vi "Command (read) - RL.vi"(7 "timeout ms (100)":i32=100, 8 "error in (no error)":errorcluster, 9 "Register":string, 10 "IP":string, 11 "connection ID in":refnum<k16>) -> (0 "error out":errorcluster, 2 "Register Value":string, 3 "connection ID out":refnum<k16>)   [LabVIEW 2016, in "SMD-7615.lvlib" / "eSCL.lvlib"]
doc: "RL - Register Load - immediate\nSets a data register to the given immediate data value. The data value is checked and stored as a Long word. When setting a Short-word register with the given Long-word data value only the lower word of the Long value is used."
uses:
  eSCL.lvlib
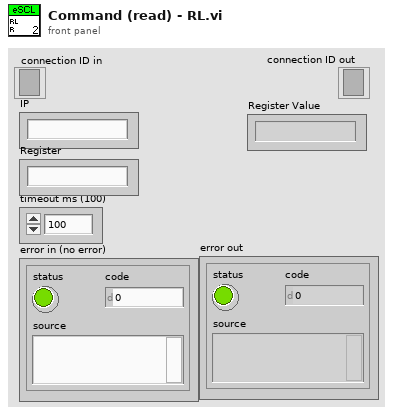
[diagram p1: front panel]
types:
  T1 = typedef "SMD-7615.lvlib/eSCL.lvlib/UDP Received Data.ctl" = cluster{"Received String":string, "eSCL Cmd":string, "Data":string}
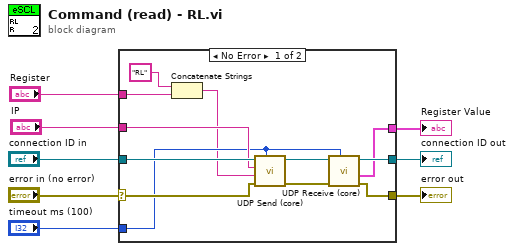
[diagram p0: block diagram]
diagram:
  n1 = case shown="No Error" "error in (no error)" {
    selector: "error in (no error)" -> [w16 w21]
    tunnel: "connection ID in" -> [w15 w22]
    tunnel: [w18 w22] -> w6
    tunnel: [w17 w21] -> w5
    tunnel: "IP" -> [w14 _]
    tunnel: "timeout ms (100)" -> [w13 _]
    tunnel: [w9 _] -> w2
    tunnel: "Register" -> [w11 _]
    frame No Error {
      n2 = Concatenate Strings("RL" ("Data"), w11) -> (w10:string)
      n3 = call "UDP Send (core).vi"("timeout ms (100)"=w13, "error in (no error)"=w16, "Data"=w10, "IP"=w14, "connection ID in"=w15) -> ("error out"=w20:errorcluster, "connection ID out"=w19:refnum<k16>)  [unwired: 5 in]
      n4 = call "UDP Receive (core).vi"("timeout ms (100)"=w13, "error in (no error)"=w20, "connection ID in"=w19) -> ("error out"=w17:errorcluster, "Received Data"=w9:T1, "connection ID out"=w18:refnum<k16>)  [unwired: 5 in, 1 out]
    }
    frame Error {
    }
  }
  "connection ID out" <- w6
  "error out" <- w5
  "Register Value" <- w2
